vi "get channel handle - by device controller index.vi"(7 "device type":T1=enum."LAN", 8 "error in (no error)":errorcluster, 10 "ip (\"\")":string, 11 "controller number(0)":u32) -> (0 "error out":errorcluster, 3 "channel handle":u16 format="%x")   [LabVIEW 2024, in "atsj peakcan basic.lvlib"]
doc: "Gets a bus channel handle for a given <b>device type </b>'s <b>controller number</b>. For LAN devices, an IP address can also be provided."
uses:
  atsj peakcan basic.lvlib
  device type.ctl
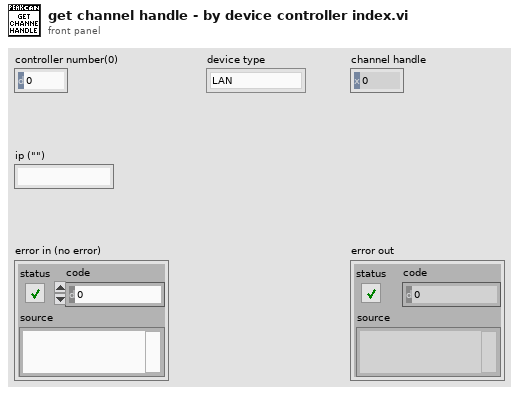
[diagram p1: front panel]
types:
  T1 = typedef "atsj peakcan basic.lvlib/device type.ctl" = enum8{"ISA", "DNG", "PCI", "USB", "PCC", "LAN"}
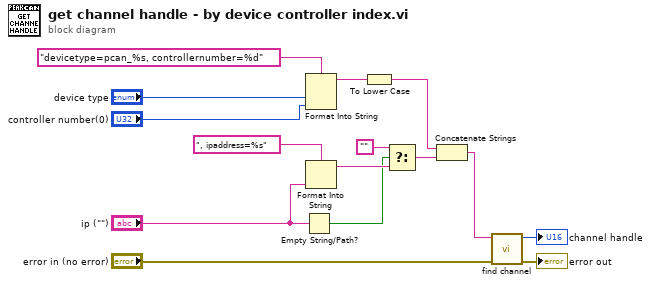
[diagram p0: block diagram]
diagram:
  n1 = Empty String/Path?(string/path="ip (\"\")") -> (empty?=w2:bool)
  n2 = Format Into String(format string="devicetype=pcan_%s, controllernumber=%d", "device type", "controller number(0)") -> (resulting string=w13:string)  [unwired: 2 in, 1 out]
  n3 = Format Into String(format string=", ipaddress=%s", "ip (\"\")") -> (resulting string=w4:string)  [unwired: 2 in, 1 out]
  n4 = To Lower Case(string=w13) -> (all lower case string=w6:string)
  n5 = Select(t="", s=w2, f=w4) -> (s? t:f=w3:string)
  n6 = Concatenate Strings(w6, w3) -> (w1:string)
  n7 = call "find channel.vi"("error in (no error)"="error in (no error)", "lookup string"=w1) -> ("error out"=→"error out":errorcluster, "channel handle"=→"channel handle":u16)  [unwired: 8 in]
